vi "FTW-ERR-Construct.vi"(7 "Status":bool, 9 "Error Code":i32, 11 "Error Message":string, 13 "Source Level":i32 caption="Source Level (0 = This VI's caller)") -> (15 "error out":errorcluster)   [LabVIEW 2018]
doc: "Constructs a new error from status, code, and string"
panel:
  # "Inputs"
  # "Outputs"
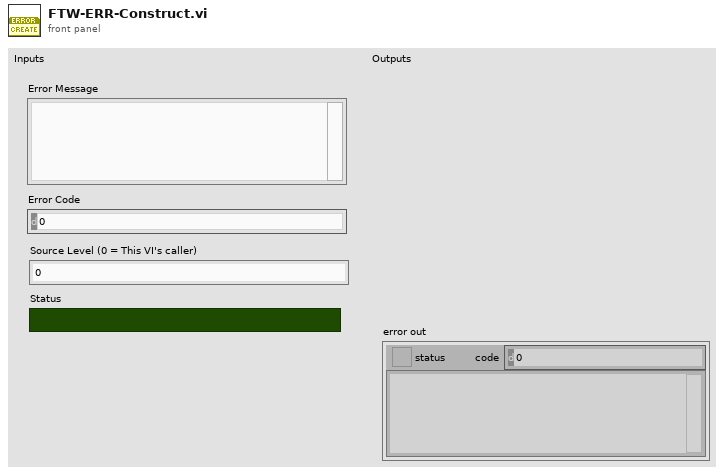
[diagram p1: front panel]
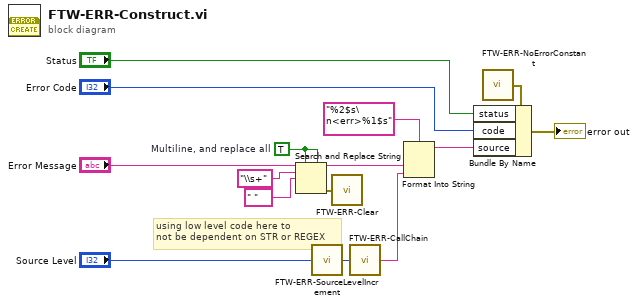
[diagram p0: block diagram]
diagram:
  w8 = TRUE  # Multiline, and replace all
  # "using low level code here to\nnot be dependent on STR or REGEX"
  n1 = Search and Replace String(replace all?=w8, multiline?=w8, input string="Error Message", search string="\\s+" ("String"), replace string=" " ("String")) -> (result string=w7:string, error out=w4:errorcluster)  [unwired: 3 in, 2 out]
  n2 = call "FTW-ERR-SourceLevelIncrement.vi"("SourceLevelIn"="Source Level") -> ("SourceLevelOut"=w1:i32)
  n3 = call "FTW-ERR-Clear.vi"("error to snuff"=w4) -> ()  [unwired: 1 out]
  n4 = call "FTW-ERR-CallChain.vi"("Source Level"=w1) -> ("Call Chain"=w9:string)
  n5 = Format Into String(format string="%2$s\n<err>%1$s", w7, w9) -> (resulting string=w11:string)  [unwired: 2 in, 1 out]
  n6 = call "FTW-ERR-NoErrorConstant.vi"() -> ("no error"=w10:errorcluster)
  n7 = Bundle By Name(cluster=w10, "status"="Status", "code"="Error Code", "source"=w11) -> (→"error out":errorcluster)
